vi "Receiver_3.vi"() -> ()   [LabVIEW 2013]
uses:
  <vilib>/imath/engines/lvmath/Plug In/_Char/NIMS_CH_character datatype.ctl
  <vilib>/imath/engines/lvmath2/RunTimeEngine/NodeEndStatement/NIMS_NodeEndStatement_Output.vi
  <instcachedir>/0/NIMS_NodeEndStatement_Output_53EC0D466D134D7ABD903AC30B43404B.lvgen/NIMS_NodeEndStatement_Output_53EC0D466D134D7ABD903AC30B43404B_005.vi
  <vilib>/imath/engines/lvmath2/RunTimeEngine/ErrorHandling/NIMS_Finalize Error.vi
  <vilib>/imath/engines/lvmath2/RunTimeEngine/Managers/WorkSpace/UID Generator.vi
  <vilib>/imath/engines/lvmath2/RunTimeEngine/Managers/SymbolTable/Clear UID.vi
  <instcachedir>/0/NIMS_NodeEndStatement_Output_53EC0D466D134D7ABD903AC30B43404B.lvgen/NIMS_NodeEndStatement_Output_53EC0D466D134D7ABD903AC30B43404B_011.vi
  <instcachedir>/0/NIMS_NodeEndStatement_Output_53EC0D466D134D7ABD903AC30B43404B.lvgen/NIMS_NodeEndStatement_Output_53EC0D466D134D7ABD903AC30B43404B_000.vi
  <vilib>/imath/engines/lvmath2/RunTimeEngine/BuiltInFunctions/close/NIMS_close(Enums).vi
  LabVIEW Data/MathScriptVIs/MCStatic_31879994332_6309011b735c7d3bdc345e9dbe068425.vi
  <instcachedir>/0/MCStatic_31879994332_6309011b735c7d3bdc345e9dbe068425_26C83AF4E6B94C66802D7F534C05881C.lvgen/MCStatic_31879994332_6309011b735c7d3bdc345e9dbe068425_26C83AF4E6B94C66802D7F534C05881C_000.vi
  <vilib>/imath/engines/lvmath2/RunTimeEngine/BuiltInFunctions/numelements/NIMS_numelements.vi
  <instcachedir>/0/NIMS_numelements_A776DA77F73142F68C2F209B523114C5.lvgen/NIMS_numelements_A776DA77F73142F68C2F209B523114C5_003.vi
  LabVIEW Data/MathScriptVIs/MCStatic_31879994332_e0c6d33342fcfeb52dca76011519375f.vi
  <instcachedir>/0/MCStatic_31879994332_e0c6d33342fcfeb52dca76011519375f_339AF80C0AAC43069D5B64E593FFC926.lvgen/MCStatic_31879994332_e0c6d33342fcfeb52dca76011519375f_339AF80C0AAC43069D5B64E593FFC926_000.vi
  <vilib>/imath/engines/lvmath2/RunTimeEngine/BuiltInFunctions/imag/NIMS_imag(Complex).vi
  <instcachedir>/0/NIMS_imag(Complex)_3180D40D00C843A49C2B33397F857BF3.lvgen/NIMS_imag(Complex)_3180D40D00C843A49C2B33397F857BF3_002.vi
  <vilib>/imath/engines/lvmath2/RunTimeEngine/BuiltInFunctions/figure/NIMS_figure(I32).vi
  <vilib>/imathl/engines/lvmath/Functions/Error Handling/Create Error.vi
  <vilib>/imath/engines/lvmath/Plug In/_Char/NIMS_CH_Character RV to String.vi
  <vilib>/imath/engines/lvmath2/RunTimeEngine/IndexRead/NIMS V(R2).vi
  <instcachedir>/0/NIMS V(R2)_C76619605A0E4E9F8B2FA9389712AC47.lvgen/NIMS V(R2)_C76619605A0E4E9F8B2FA9389712AC47_000.vi
  <vilib>/imath/engines/lvmath2/RunTimeEngine/ArithmeticOperatorToken/NIMS_ArithmeticOperator_plus.vi
  <instcachedir>/0/NIMS_ArithmeticOperator_plus_8A46DAFC24D445C9B2C97B626139369E.lvgen/NIMS_ArithmeticOperator_plus_8A46DAFC24D445C9B2C97B626139369E_005.vi
  <vilib>/imath/engines/lvmath2/RunTimeEngine/BuiltInFunctions/plot/NIMS_plot(G, Str).vi
  <instcachedir>/0/NIMS_plot(G, Str)_30D49D8623E0484DBD39D394DDFCBE95.lvgen/NIMS_plot(G, Str)_30D49D8623E0484DBD39D394DDFCBE95_001.vi
  <vilib>/imath/engines/lvmath2/RunTimeEngine/ErrorHandling/NIMS_Create Error From Enums.vi
  <vilib>/imath/engines/lvmath2/RunTimeEngine/BuiltInFunctions/grid/NIMS_grid(Enums).vi
  <vilib>/imath/engines/lvmath/Plug In/_Char/NIMS_CH_Character 1D to U8 1D.vi
  <vilib>/imath/engines/lvmath2/RunTimeEngine/BuiltInFunctions/plot/NIMS_plot(G, Arb).vi
  <instcachedir>/0/NIMS_plot(G, Arb)_C3943409FB664E118D06A85D9C4CA97C.lvgen/NIMS_plot(G, Arb)_C3943409FB664E118D06A85D9C4CA97C_000.vi
  <vilib>/imath/engines/lvmath2/RunTimeEngine/BuiltInFunctions/hold/NIMS_hold(Enums).vi
  <vilib>/imath/engines/lvmath2/RunTimeEngine/VariableToken/NIMS_VariableToken_CondDefined.vi
  <instcachedir>/0/NIMS_VariableToken_CondDefined_9DC5CEC47F8146B087FA2781C705B229.lvgen/NIMS_VariableToken_CondDefined_9DC5CEC47F8146B087FA2781C705B229_003.vi
  <vilib>/imath/engines/lvmath/Functions/Error Handling/MergeErrorsWrapper.vi
  <instcachedir>/0/NIMS_NodeEndStatement_Output_53EC0D466D134D7ABD903AC30B43404B.lvgen/NIMS_NodeEndStatement_Output_53EC0D466D134D7ABD903AC30B43404B_001.vi
  LabVIEW Data/MathScriptVIs/MCStatic_31879994332_4a1719067c7d5a83f01437ef7afed563.vi
  <instcachedir>/0/MCStatic_31879994332_4a1719067c7d5a83f01437ef7afed563_594FF1B2330943F592931CE525BA3D62.lvgen/MCStatic_31879994332_4a1719067c7d5a83f01437ef7afed563_594FF1B2330943F592931CE525BA3D62_001.vi
  <vilib>/imath/engines/lvmath2/RunTimeEngine/BuiltInFunctions/crosscorr/NIMS_crosscorr(GM,GM,Str).vi
  <instcachedir>/0/NIMS_crosscorr(GM,GM,Str)_C0B084FC02374B5995655F2C6E77F5A9.lvgen/NIMS_crosscorr(GM,GM,Str)_C0B084FC02374B5995655F2C6E77F5A9_001.vi
  <vilib>/imath/engines/lvmath2/RunTimeEngine/BuiltInFunctions/abs/NIMS_abs(signed).vi
  <instcachedir>/0/NIMS_abs(signed)_C4FCB8E6058B49B797C7C8D53CA5F6EC.lvgen/NIMS_abs(signed)_C4FCB8E6058B49B797C7C8D53CA5F6EC_003.vi
  <instcachedir>/0/NIMS_plot(G, Str)_30D49D8623E0484DBD39D394DDFCBE95.lvgen/NIMS_plot(G, Str)_30D49D8623E0484DBD39D394DDFCBE95_004.vi
  <instcachedir>/0/NIMS_plot(G, Str)_30D49D8623E0484DBD39D394DDFCBE95.lvgen/NIMS_plot(G, Str)_30D49D8623E0484DBD39D394DDFCBE95_005.vi
  <instcachedir>/0/NIMS_crosscorr(GM,GM,Str)_C0B084FC02374B5995655F2C6E77F5A9.lvgen/NIMS_crosscorr(GM,GM,Str)_C0B084FC02374B5995655F2C6E77F5A9_000.vi
  <instcachedir>/0/NIMS_abs(signed)_C4FCB8E6058B49B797C7C8D53CA5F6EC.lvgen/NIMS_abs(signed)_C4FCB8E6058B49B797C7C8D53CA5F6EC_005.vi
  <vilib>/imath/engines/lvmath2/RunTimeEngine/BuiltInFunctions/max/1 input/NIMS_max(RM).vi
  <instcachedir>/0/NIMS_max(RM)_95FF4207DE024F99B69DE66176218BBE.lvgen/NIMS_max(RM)_95FF4207DE024F99B69DE66176218BBE_000.vi
  <vilib>/imath/engines/lvmath2/RunTimeEngine/BuiltInFunctions/length/NIMS_length(GV).vi
  <instcachedir>/0/NIMS_length(GV)_08A3D13377FD4E4B96F5795FBF3698FA.lvgen/NIMS_length(GV)_08A3D13377FD4E4B96F5795FBF3698FA_001.vi
  <vilib>/imath/engines/lvmath2/RunTimeEngine/BuiltInFunctions/length/NIMS_length(GM).vi
  <instcachedir>/0/NIMS_length(GM)_47CEC356FCE0482D9BA47DC61C99F2C7.lvgen/NIMS_length(GM)_47CEC356FCE0482D9BA47DC61C99F2C7_005.vi
  <instcachedir>/0/NIMS V(R2)_C76619605A0E4E9F8B2FA9389712AC47.lvgen/NIMS V(R2)_C76619605A0E4E9F8B2FA9389712AC47_001.vi
  <vilib>/imath/engines/lvmath2/RunTimeEngine/RunTimeType/NIMS_RunTimeType_From StrictType (excl LVString).vi
  <instcachedir>/0/NIMS_RunTimeType_From StrictType (excl LVString)_4DEE718D6EB74582AA20236969C084FC.lvgen/NIMS_RunTimeType_From StrictType (excl LVString)_4DEE718D6EB74582AA20236969C084FC_000.vi
  <vilib>/imath/engines/lvmath2/RunTimeEngine/LocalVariableDefStatement/MC_LocalVariableDefStatement_Display.vi
  <vilib>/imath/engines/lvmath2/RunTimeEngine/BuiltInFunctions/linramp/NIMS_linramp.vi
  <instcachedir>/0/NIMS_abs(signed)_C4FCB8E6058B49B797C7C8D53CA5F6EC.lvgen/NIMS_abs(signed)_C4FCB8E6058B49B797C7C8D53CA5F6EC_006.vi
  <vilib>/imath/engines/lvmath2/RunTimeEngine/BuiltInFunctions/max/1 input/NIMS_max(RV).vi
  <instcachedir>/0/NIMS_max(RV)_237633DB1D604D5BA7001287DF3C7957.lvgen/NIMS_max(RV)_237633DB1D604D5BA7001287DF3C7957_000.vi
  <vilib>/imath/engines/lvmath2/RunTimeEngine/BuiltInFunctions/zeros/NIMS_V=zeros(I32,I32).vi
  <vilib>/imath/engines/lvmath2/RunTimeEngine/RangeToken/NIMS_Range_R2 - Integer.vi
  <instcachedir>/0/NIMS_Range_R2 - Integer_C51C130E5EA5464EA148B28CDAB9615A.lvgen/NIMS_Range_R2 - Integer_C51C130E5EA5464EA148B28CDAB9615A_000.vi
  <vilib>/imath/engines/lvmath2/RunTimeEngine/CommandStatement/MC_CommandStatement_break.vi
  <vilib>/imath/engines/lvmath2/RunTimeEngine/IndexRead/NIMS V(S).vi
  <instcachedir>/0/NIMS V(S)_0488751826AF41519A22953C041130DC.lvgen/NIMS V(S)_0488751826AF41519A22953C041130DC_005.vi
  <instcachedir>/0/NIMS_abs(signed)_C4FCB8E6058B49B797C7C8D53CA5F6EC.lvgen/NIMS_abs(signed)_C4FCB8E6058B49B797C7C8D53CA5F6EC_002.vi
  LabVIEW Data/MathScriptVIs/MCStatic_31879994332_56053b3087a32285ab019b20dd55a053.vi
  <instcachedir>/0/MCStatic_31879994332_56053b3087a32285ab019b20dd55a053_ABD68300304F468FBDE6379C6945ADEA.lvgen/MCStatic_31879994332_56053b3087a32285ab019b20dd55a053_ABD68300304F468FBDE6379C6945ADEA_000.vi
  <vilib>/imath/engines/lvmath2/RunTimeEngine/IndexReplace/NIMS V(S)=S.vi
  <instcachedir>/0/NIMS V(S)=S_66A18068148B4981A312229A93EA5C06.lvgen/NIMS V(S)=S_66A18068148B4981A312229A93EA5C06_001.vi
  LabVIEW Data/MathScriptVIs/MCStatic_31879994332_59775c3ea1da542a74dd2e471b583196.vi
  <instcachedir>/0/MCStatic_31879994332_59775c3ea1da542a74dd2e471b583196_003FAE1D6247465EB97E783626A83D88.lvgen/MCStatic_31879994332_59775c3ea1da542a74dd2e471b583196_003FAE1D6247465EB97E783626A83D88_001.vi
  <instcachedir>/0/NIMS V(S)=S_66A18068148B4981A312229A93EA5C06.lvgen/NIMS V(S)=S_66A18068148B4981A312229A93EA5C06_000.vi
  <instcachedir>/0/NIMS V(S)_0488751826AF41519A22953C041130DC.lvgen/NIMS V(S)_0488751826AF41519A22953C041130DC_000.vi
  <instcachedir>/0/NIMS_plot(G, Str)_30D49D8623E0484DBD39D394DDFCBE95.lvgen/NIMS_plot(G, Str)_30D49D8623E0484DBD39D394DDFCBE95_000.vi
  <vilib>/imath/engines/lvmath2/RunTimeEngine/BuiltInFunctions/title/NIMS_title.vi
  <instcachedir>/0/NIMS_NodeEndStatement_Output_53EC0D466D134D7ABD903AC30B43404B.lvgen/NIMS_NodeEndStatement_Output_53EC0D466D134D7ABD903AC30B43404B_012.vi
  <vilib>/imath/engines/lvmath2/RunTimeEngine/VariableToken/NIMS_VariableToken_CondDefinedDefinedByReplace.vi
  <instcachedir>/0/NIMS_VariableToken_CondDefinedDefinedByReplace_D162CFFC24174562A9FEA619A91E1A56.lvgen/NIMS_VariableToken_CondDefinedDefinedByReplace_D162CFFC24174562A9FEA619A91E1A56_002.vi
  <vilib>/imath/engines/lvmath2/RunTimeEngine/IndexRead/NIMS M(S).vi
  <instcachedir>/0/NIMS M(S)_B826C018497E4940AE96BD27B540B6FB.lvgen/NIMS M(S)_B826C018497E4940AE96BD27B540B6FB_004.vi
  <instcachedir>/0/NIMS_VariableToken_CondDefined_9DC5CEC47F8146B087FA2781C705B229.lvgen/NIMS_VariableToken_CondDefined_9DC5CEC47F8146B087FA2781C705B229_004.vi
  <vilib>/imath/engines/lvmath2/RunTimeEngine/BuiltInFunctions/min/1 input/NIMS_min(RV).vi
  <instcachedir>/0/NIMS_min(RV)_EE2DD3E2888846108C5160A664B67832.lvgen/NIMS_min(RV)_EE2DD3E2888846108C5160A664B67832_000.vi
  <vilib>/imath/engines/lvmath2/RunTimeEngine/IndexRead/NIMS M(S,S).vi
  <instcachedir>/0/NIMS M(S,S)_AC51E74150A542F7991B9634C66F3096.lvgen/NIMS M(S,S)_AC51E74150A542F7991B9634C66F3096_003.vi
  <vilib>/imath/engines/lvmath2/RunTimeEngine/RowToken/NIMS_RowToken_M_SorRV.vi
  <instcachedir>/0/NIMS_RowToken_M_SorRV_6464340A296F47B6970F468C8541F43A.lvgen/NIMS_RowToken_M_SorRV_6464340A296F47B6970F468C8541F43A_001.vi
  <vilib>/imath/engines/lvmath2/RunTimeEngine/IndexReplace/NIMS M($,S)=M.vi
  <instcachedir>/0/NIMS M($,S)=M_9C9B00E4835C49429FADE7516194B3E0.lvgen/NIMS M($,S)=M_9C9B00E4835C49429FADE7516194B3E0_002.vi
  <vilib>/imath/engines/lvmath2/RunTimeEngine/IndexReplace/NIMS M($,S)=V.vi
  <instcachedir>/0/NIMS M($,S)=V_D41FDDDB142B47FCA5EF37B60D4970ED.lvgen/NIMS M($,S)=V_D41FDDDB142B47FCA5EF37B60D4970ED_001.vi
  <vilib>/imath/engines/lvmath2/RunTimeEngine/ArithmeticOperatorToken/NIMS_ArithmeticOperator_minus.vi
  <instcachedir>/0/NIMS_ArithmeticOperator_minus_5462A7974F41415E96B34B7C9D041F4F.lvgen/NIMS_ArithmeticOperator_minus_5462A7974F41415E96B34B7C9D041F4F_001.vi
  <vilib>/imath/engines/lvmath2/RunTimeEngine/BuiltInFunctions/sum/NIMS_sum(GM,Sca).vi
  <instcachedir>/0/NIMS_sum(GM,Sca)_6844B20AF95244A89239C08EE60A7865.lvgen/NIMS_sum(GM,Sca)_6844B20AF95244A89239C08EE60A7865_001.vi
  <vilib>/imath/engines/lvmath2/RunTimeEngine/BuiltInFunctions/crosscorr/NIMS_crosscorr(GM,Sca,Str).vi
  <instcachedir>/0/NIMS_crosscorr(GM,Sca,Str)_6201EFE436AF4A49A2EDE7F536F431B0.lvgen/NIMS_crosscorr(GM,Sca,Str)_6201EFE436AF4A49A2EDE7F536F431B0_000.vi
  <instcachedir>/0/NIMS_length(GV)_08A3D13377FD4E4B96F5795FBF3698FA.lvgen/NIMS_length(GV)_08A3D13377FD4E4B96F5795FBF3698FA_002.vi
  MATLAB_func/RX_RRC_filtering.m
  MATLAB_func/rtrcpulse.m
  MATLAB_func/gardner_symbol_recovery.m
  MATLAB_func/b2_16qam.m
  MATLAB_func/frequency_synchronisation_sample.m
  MATLAB_func/phase_synchronisation_sample.m
  <vilib>/imath/engines/lvmath2/RunTimeEngine/Managers/SymbolTable/NIMS_WorkSpace.lvlib
panel:
  out "error":dbl[](array[numeric])
  out "signal_out":i32[][](array[numeric])
  out "Real 2":dbl
  out "N":i32
  out "L":i32
  out "Symbols 4":cdb[](graph)
  out "1-D Array of Complex":cdb[](array[numeric])
  out "wave array":cdb[](array[numeric])
  out "sym array":cdb[](array[numeric])
  out "Symbols 3":cdb[](graph)
  out "1-D Array of Complex 4":cdb[](array[numeric])
  out "Real":dbl
  out "Waveform Chart":dbl[](graph)
  out "First Start":dbl(graph)
  out "Symbols 1":cdb[](graph)
  out "Symbols 2":cdb[](graph)
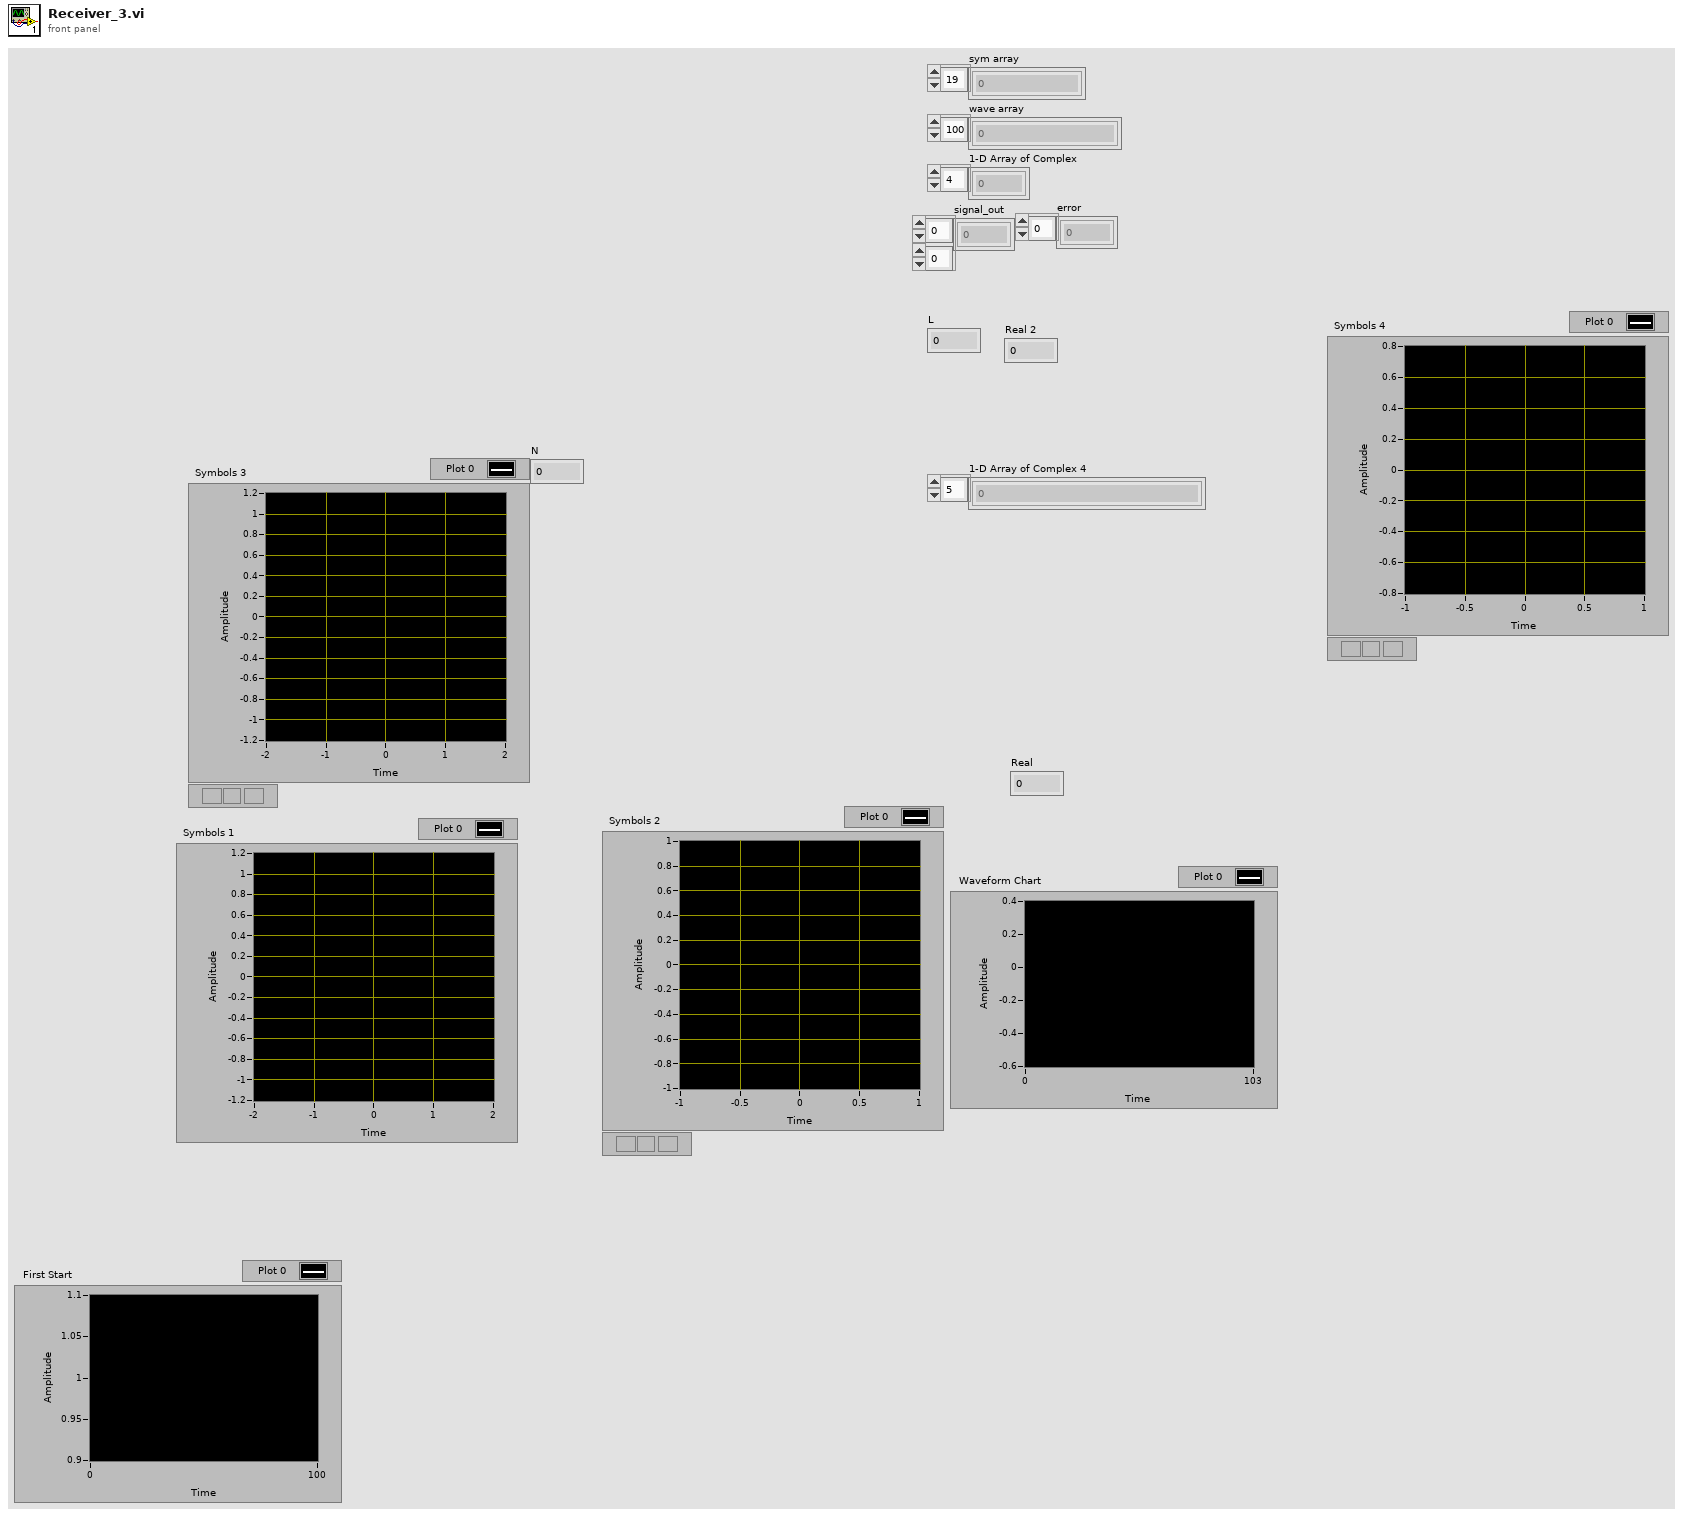
[diagram p1: front panel]
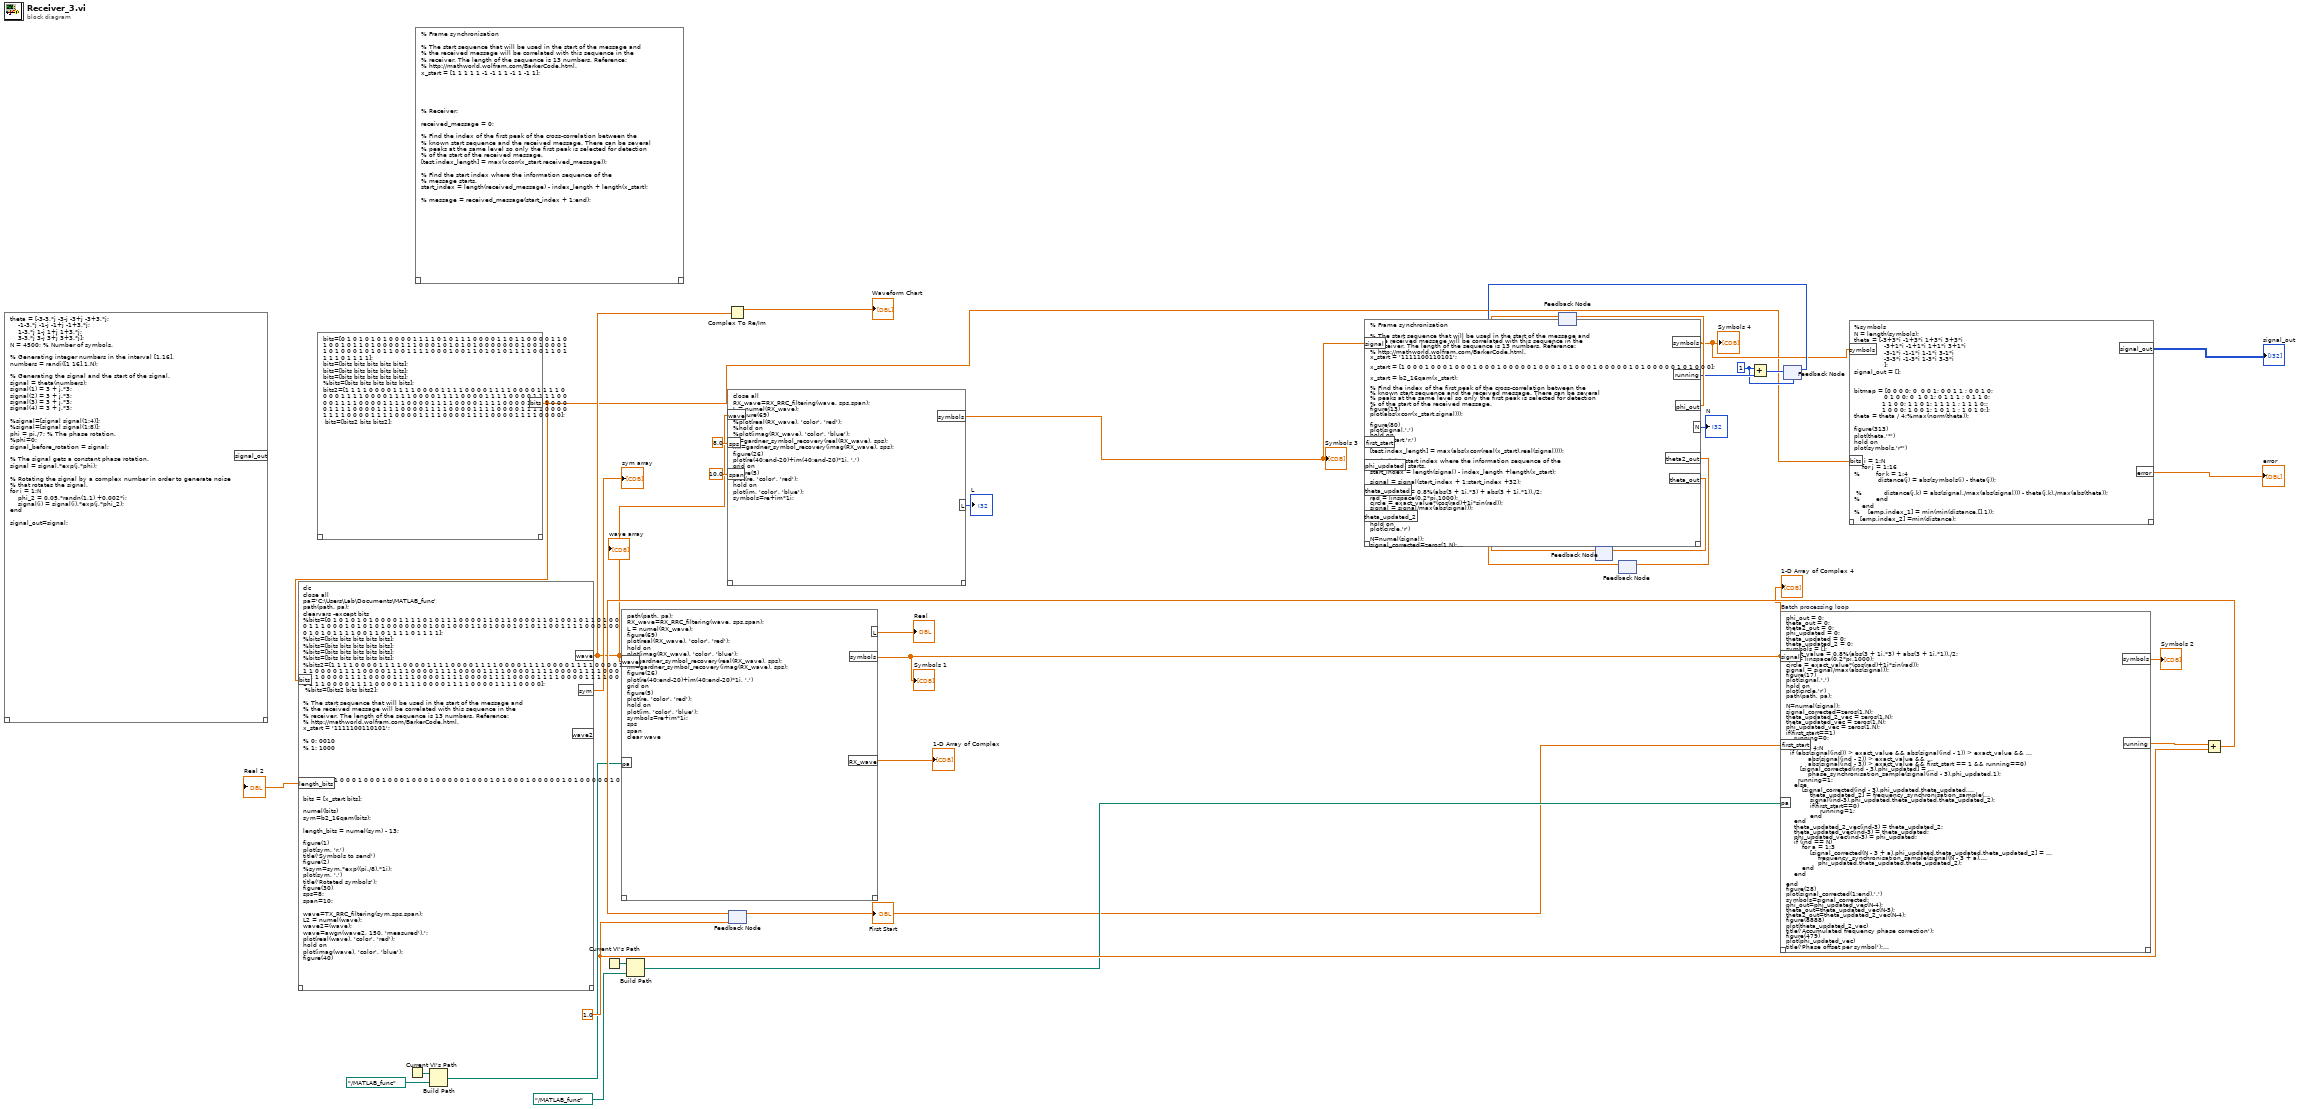
[diagram p0: block diagram]
diagram:
  w9 = 1 ("x")
  w36 = 1.0
  n1 = script code="theta = [-3-3.*j -3-j -3+j -3+3.*j;\n    -1-3.*j -1-j -1+j -1+3.*j;\n    1-3.*j 1-j 1+j 1+3.*j;\n    3-3.*j 3-j 3+j 3+3.*j];\nN = 4500; % Number of symbols.\n\n% Generating integer numbers in the interval [1,16].\nnumbers = randi([1 16],1,N);\n\n% Generating the signal and the start of the signal.\nsignal = theta(numbers);\nsignal(1) = 3 + j.*3;\nsignal(2) = 3 + j.*3;\nsignal(3) = 3 + j.*3;\nsignal(4) = 3 + j.*3;\n\n%signal=[signal signal(1:4)];\n%signal=[signal signal(1:8)];\nphi = pi./7; % The phase rotation.\n%phi=0;\nsignal_before_rotation = signal;\n\n% The signal gets a constant phase rotation.\nsignal = signal.*exp(j.*phi);\n\n% Rotating the signal by a complex number in order to generate noise\n% that rotates the signal.\nfor i = 1:N\n    phi_2 = 0.05.*randn(1,1) +0.002*i;\n    signal(i) = signal(i).*exp(j.*phi_2);\nend\n\nsignal_out=signal;"() -> ()  [unwired: 1 in, 2 out]
  n2 = mathscript code="bits=[0 1 0 1 0 1 0 1 0 0 0 0 1 1 1 1 0 1 0 1 1 1 0 0 0 0 1 1 0 1 1 0 0 0 0 1 1 0 1 0 0 1 0 1 1 0 1 0 0 0 0 1 1 1 0 0 0 1 0 1 0 1 0 1 0 0 0 0 0 0 0 1 0 0 1 0 0 0 1 1 0 1 0 0 0 1 0 1 0 1 1 0 0 1 1 1 1 0 0 0 1 0 0 1 1 0 1 0 1 0 1 1 1 1 0 0 1 1 0 1 1 1 1 0 1 1 1 1];\nbits=[bits bits bits bits bits];\nbits=[bits bits bits bits bits];\nbits=[bits bits bits bits bits];\n%bits=[bits bits bits bits bits];\nbits2=[1 1 1 1 0 0 0 0 1 1 1 1 0 0 0 0 1 1 1 1 0 0 0 0 1 1 1 1 0 0 0 0 1 1 1 1 0 0 0 0 1 1 1 1 0 0 0 0 1 1 1 1 0 0 0 0 1 1 1 1 0 0 0 0 1 1 1 1 0 0 0 0 1 1 1 1 0 0 0 0 1 1 1 1 0 0 0 0 1 1 1 1 0 0 0 0 1 1 1 1 0 0 0 0 1 1 1 1 0 0 0 0 1 1 1 1 0 0 0 0 1 1 1 1 0 0 0 0 1 1 1 1 0 0 0 0 1 1 1 1 0 0 0 0 1 1 1 1 0 0 0 0 1 1 1 1 0 0 0 0 1 1 1 1 0 0 0 0 1 1 1 1 0 0 0 0 1 1 1 1 0 0 0 0 1 1 1 1 0 0 0 0 1 1 1 1 0 0 0 0]; \n bits=[bits2 bits bits2];"() -> ("bits"=w2:dbl[])  [unwired: 1 in, 1 out]
  n3 = script code="clc\nclose all\npa='C:\\Users\\Lab\\Documents\\MATLAB_func'\npath(path, pa);\nclearvars -except bits\n%bits=[0 1 0 1 0 1 0 1 0 0 0 0 1 1 1 1 0 1 0 1 1 1 0 0 0 0 1 1 0 1 1 0 0 0 0 1 1 0 1 0 0 1 0 1 1 0 1 0 0 0 0 1 1 1 0 0 0 1 0 1 0 1 0 1 0 0 0 0 0 0 0 1 0 0 1 0 0 0 1 1 0 1 0 0 0 1 0 1 0 1 1 0 0 1 1 1 1 0 0 0 1 0 0 1 1 0 1 0 1 0 1 1 1 1 0 0 1 1 0 1 1 1 1 0 1 1 1 1];\n%bits=[bits bits bits bits bits];\n%bits=[bits bits bits bits bits];\n%bits=[bits bits bits bits bits];\n%bits=[bits bits bits bits bits];\n%bits2=[1 1 1 1 0 0 0 0 1 1 1 1 0 0 0 0 1 1 1 1 0 0 0 0 1 1 1 1 0 0 0 0 1 1 1 1 0 0 0 0 1 1 1 1 0 0 0 0 1 1 1 1 0 0 0 0 1 1 1 1 0 0 0 0 1 1 1 1 0 0 0 0 1 1 1 1 0 0 0 0 1 1 1 1 0 0 0 0 1 1 1 1 0 0 0 0 1 1 1 1 0 0 0 0 1 1 1 1 0 0 0 0 1 1 1 1 0 0 0 0 1 1 1 1 0 0 0 0 1 1 1 1 0 0 0 0 1 1 1 1 0 0 0 0 1 1 1 1 0 0 0 0 1 1 1 1 0 0 0 0 1 1 1 1 0 0 0 0 1 1 1 1 0 0 0 0 1 1 1 1 0 0 0 0 1 1 1 1 0 0 0 0 1 1 1 1 0 0 0 0]; \n %bits=[bits2 bits bits2];\n\n% The start sequence that will be used in the start of the message and\n% the received message will be correlated with this sequence in the \n% receiver. The length of the sequence is 13 numbers. Reference: \n% http://mathworld.wolfram.com/BarkerCode.html.\nx_start = '1111100110101';\n\n% 0: 0010\n% 1: 1000\n\n\n\n\nx_start = [1 0 0 0 1 0 0 0 1 0 0 0 1 0 0 0 1 0 0 0 0 0 1 0 0 0 1 0 1 0 0 0 1 0 0 0 0 0 1 0 1 0 0 0 0 0 1 0 1 0 0 0];\n\nbits = [x_start bits];\n\nnumel(bits)\nsym=b2_16qam(bits);\n\nlength_bits = numel(sym) - 13;\n\nfigure(1)\nplot(sym, 'r.')\ntitle('Symbols to send')\nfigure(2)\n%sym=sym.*exp((pi./8).*1i);\nplot(sym, '.')\ntitle('Rotated symbols');\nfigure(30)\nsps=8;\nspan=10;\n\nwave=TX_RRC_filtering(sym,sps,span);\nL2 = numel(wave);\nwave2=(wave);\nwave=awgn(wave2, 150, 'measured').';\nplot(real(wave), 'color', 'red');\nhold on\nplot(imag(wave), 'color', 'blue');\nfigure(40)"("bits"=w2) -> ("wave"=w19:cdb[], "sym"=→"sym array":cdb[], "length_bits"=→"Real 2":dbl)  [unwired: 1 in, 2 out]
  "wave array" <- w19
  n4 = Current VI's Path() -> (path=w29:path)
  n5 = mathscript code="% Frame synchronisation\n\n% The start sequence that will be used in the start of the message and\n% the received message will be correlated with this sequence in the \n% receiver. The length of the sequence is 13 numbers. Reference: \n% http://mathworld.wolfram.com/BarkerCode.html.\nx_start = [1 1 1 1 1 -1 -1 1 1 -1 1 -1 1];\n\n\n\n\n\n% Receiver:\n\nreceived_message = 0;\n\n% Find the index of the first peak of the cross-correlation between the \n% known start sequence and the received message. There can be several \n% peaks at the same level so only the first peak is selected for detection \n% of the start of the received message.\n[test,index_length] = max(xcorr(x_start,received_message));\n\n% Find the start index where the information sequence of the \n% message starts.\nstart_index = length(received_message) - index_length + length(x_start);\n\n% message = received_message(start_index + 1:end);"() -> ()  [unwired: 1 in, 1 out]
  n6 = Build Path(base path=w29, name or relative path=path "../MATLAB_func") -> (appended path=w30:path)
  n7 = Current VI's Path() -> (path=w33:path)
  n8 = script code="path(path, pa);\nRX_wave=RX_RRC_filtering(wave, sps,span);\nL = numel(RX_wave);\nfigure(69)\nplot(real(RX_wave), 'color', 'red');\nhold on\nplot(imag(RX_wave), 'color', 'blue');\nre=gardner_symbol_recovery(real(RX_wave), sps);\nim=gardner_symbol_recovery(imag(RX_wave), sps);\nfigure(26)\nplot(re(40:end-20)+im(40:end-20)*1i, '.')\ngrid on\nfigure(5)\nplot(re, 'color', 'red');\nhold on\nplot(im, 'color', 'blue');\nsymbols=re+im*1i;\nsps\nspan\nclear wave"("wave"=w19, "pa"=w30) -> ("symbols"=w22:cdb[], "L"=→"Real":dbl, "RX_wave"=→"1-D Array of Complex":cdb[])  [unwired: 1 in, 1 out]
  "Symbols 1" <- w22
  "1-D Array of Complex 4" <- w22
  n9 = Build Path(base path=w33, name or relative path=path "../MATLAB_func") -> (appended path=w34:path)
  n10 = mathscript code="close all\nRX_wave=RX_RRC_filtering(wave, sps,span);\nL = numel(RX_wave);\n%figure(69)\n%plot(real(RX_wave), 'color', 'red');\n%hold on\n%plot(imag(RX_wave), 'color', 'blue');\nre=gardner_symbol_recovery(real(RX_wave), sps);\nim=gardner_symbol_recovery(imag(RX_wave), sps);\nfigure(26)\nplot(re(40:end-20)+im(40:end-20)*1i, '.')\ngrid on\nfigure(5)\nplot(re, 'color', 'red');\nhold on\nplot(im, 'color', 'blue');\nsymbols=re+im*1i;"("wave"=w19, "sps"=8.0, "span"=10.0) -> ("symbols"=w18:cdb[], "L"=→"L":i32)  [unwired: 1 in, 1 out]
  "Symbols 3" <- w18
  n11 = Complex To Re/Im(x + iy=w19) -> (x=→"Waveform Chart":dbl[])  [unwired: 1 out]
  n12 = feedback #1(w36) -> (w25:dbl)
  "First Start" <- w25
  n13 = feedback #2() -> (w12:dbl)  [unwired: 1 in]
  n14 = feedback #3() -> (w16:dbl)  [unwired: 1 in]
  n15 = feedback #4() -> (w14:dbl)  [unwired: 1 in]
  n16 = script code="phi_out = 0;\ntheta_out = 0;\ntheta2_out = 0;\nphi_updated = 0;\ntheta_updated = 0;\ntheta_updated_2 = 0;\nsymbols = [];\nexact_value = 0.8%(abs(3 + 1i.*3) + abs(3 + 1i.*1))./2;\nrad = linspace(0,2*pi,1000);\ncircle = exact_value*(cos(rad)+1i*sin(rad));\nsignal = signal/max(abs(signal));\nfigure(17)\nplot(signal,'.')\nhold on\nplot(circle,'r')\npath(path, pa);\n\nN=numel(signal);\nsignal_corrected=zeros(1,N);\ntheta_updated_2_vec = zeros(1,N);\ntheta_updated_vec = zeros(1,N);\nphi_updated_vec = zeros(1,N);\nif(first_start==1)\n    running=0;\nend\nfor ind= 4:N\n  if (abs(signal(ind)) > exact_value && abs(signal(ind - 1)) > exact_value && ...\n           abs(signal(ind - 2)) > exact_value && ...\n           abs(signal(ind - 3)) > exact_value && first_start == 1 && running==0)\n       [signal_corrected(ind - 3),phi_updated] = ...\n           phase_synchronisation_sample(signal(ind - 3),phi_updated,1);\n      running=1;\n    else\n        [signal_corrected(ind - 3),phi_updated,theta_updated,...\n            theta_updated_2] = frequency_synchronisation_sample(...\n            signal(ind-3),phi_updated,theta_updated,theta_updated_2);\n            if(first_start==0)\n                 running=1;\n            end\n    end\n    theta_updated_2_vec(ind-3) = theta_updated_2;\n    theta_updated_vec(ind-3) = theta_updated;\n    phi_updated_vec(ind-3) = phi_updated;\n    if (ind == N)\n        for a = 1:3\n            [signal_corrected(N - 3 + a),phi_updated,theta_updated,theta_updated_2] = ...\n                frequency_synchronisation_sample(signal(N - 3 + a),...\n                phi_updated,theta_updated,theta_updated_2);\n        end\n    end\n\nend\nfigure(28)\nplot(signal_corrected(1:end),'.')\nsymbols=signal_corrected;\nphi_out=phi_updated_vec(N-4);\ntheta_out=theta_updated_vec(N-5);\ntheta2_out=theta_updated_2_vec(N-4);\nfigure(8888)\nplot(theta_updated_2_vec)\ntitle('Accumulated frequency phase correction');\nfigure(479)\nplot(phi_updated_vec)\ntitle('Phase offset per symbol');\nhold off\nfigure(1337)\nplot(symbols(100:end-20),'.')\nclear all\n% clearvars -except symbols running phi_out theta_out theta2_out" "Batch processing loop"("signal"=w22, "first_start"=w25, "pa"=w34) -> ("symbols"=→"Symbols 2":cdb[], "running"=w31:dbl)  [unwired: 1 in, 1 out]
  n17 = feedback #5(w9) -> (w8:i32)
  n18 = mathscript code="% Frame synchronisation\n\n% The start sequence that will be used in the start of the message and\n% the received message will be correlated with this sequence in the \n% receiver. The length of the sequence is 13 numbers. Reference: \n% http://mathworld.wolfram.com/BarkerCode.html.\nx_start = '1111100110101';\n\nx_start = [1 0 0 0 1 0 0 0 1 0 0 0 1 0 0 0 1 0 0 0 0 0 1 0 0 0 1 0 1 0 0 0 1 0 0 0 0 0 1 0 1 0 0 0 0 0 1 0 1 0 0 0];\n\nx_start = b2_16qam(x_start);\n\n% Find the index of the first peak of the cross-correlation between the \n% known start sequence and the received message. There can be several \n% peaks at the same level so only the first peak is selected for detection \n% of the start of the received message.\nfigure(13)\nplot(abs(xcorr(x_start,signal)));\n\nfigure(80)\nplot(signal,'.')\nhold on\nplot(x_start,'r.')\n\n[test,index_length] = max(abs(xcorr(real(x_start),real(signal))));\n\n% Find the start index where the information sequence of the \n% message starts.\nstart_index = length(signal) - index_length +length(x_start);\n\nsignal = signal(start_index + 1:start_index +32);\n\nexact_value = 0.8%(abs(3 + 1i.*3) + abs(3 + 1i.*1))./2;\nrad = linspace(0,2*pi,1000);\ncircle = exact_value*(cos(rad)+1i*sin(rad));\nsignal = signal/max(abs(signal));\nfigure(17)\nplot(signal,'.')\nhold on\nplot(circle,'r')\n\nN=numel(signal);\nsignal_corrected=zeros(1,N);\ntheta_updated_2_vec = zeros(1,N);\ntheta_updated_vec = zeros(1,N);\nphi_updated_vec = zeros(1,N);\nif(first_start==1)\n    running=0;\nend\nfor ind= 4:N\n  if (abs(signal(ind)) > exact_value && abs(signal(ind - 1)) > exact_value && ...\n           abs(signal(ind - 2)) > exact_value && ...\n           abs(signal(ind - 3)) > exact_value && first_start == 1 && running==0)\n       [signal_corrected(ind - 3),phi_updated] = ...\n           phase_synchronisation_sample(signal(ind - 3),phi_updated,1);\n      running=1;\n    else\n        [signal_corrected(ind - 3),phi_updated,theta_updated,...\n            theta_updated_2] = frequency_synchronisation_sample(...\n            signal(ind-3),phi_updated,theta_updated,theta_updated_2);\n            if(first_start==0)\n                 running=1;\n            end\n    end\n    theta_updated_2_vec(ind-3) = theta_updated_2;\n    theta_updated_vec(ind-3) = theta_updated;\n    phi_updated_vec(ind-3) = phi_updated;\n    if (ind == N)\n        for a = 1:3\n            [signal_corrected(N - 3 + a),phi_updated,theta_updated,theta_updated_2] = ...\n                frequency_synchronisation_sample(signal(N - 3 + a),...\n                phi_updated,theta_updated,theta_updated_2);\n        end\n    end\n\nend\nfigure(28)\nplot(signal_corrected(1:end),'.')\nsymbols=signal_corrected;\nphi_out=phi_updated_vec(N-4);\ntheta_out=theta_updated_vec(N-5);\ntheta2_out=theta_updated_2_vec(N-4);\nfigure(8888)\nplot(theta_updated_2_vec)\ntitle('Accumulated frequency phase correction');\nfigure(479)\nplot(phi_updated_vec)\ntitle('Phase offset per symbol');\nhold off\nfigure(1337)\nplot(symbols(1000:end-20),'.')"("first_start"=w8, "signal"=w18, "phi_updated"=w12, "theta_updated"=w16, "theta_updated_2"=w14) -> ("symbols"=w4:cdb[], "running"=w11:i32, "phi_out"=w13:dbl, "theta2_out"=w15:dbl, "theta_out"=w17:dbl, "N"=→"N":i32)  [unwired: 1 in, 1 out]
  "Symbols 4" <- w4
  n19 = feedback-in #2(w13) -> ()
  n20 = feedback-in #3(w17) -> ()
  n21 = feedback-in #4(w15) -> ()
  n22 = Add(x=w9, y=w11) -> (x+y=w10:i32)
  n23 = feedback-in #5(w10) -> ()
  n24 = mathscript code="%symbols\nN = length(symbols);\ntheta = [-3+3*i -1+3*i 1+3*i 3+3*i\n               -3+1*i -1+1*i 1+1*i 3+1*i\n               -3-1*i -1-1*i 1-1*i 3-1*i\n               -3-3*i -1-3*i 1-3*i 3-3*i\n               ];\nsignal_out = [];\n\n\nbitmap = [0 0 0 0; 0  0 0 1; 0 0 1 1 ; 0 0 1 0;\n               0 1 0 0; 0  1 0 1; 0 1 1 1 ; 0 1 1 0;\n              1 1 0 0; 1 1 0 1; 1 1 1 1 ; 1 1 1 0;;\n              1 0 0 0; 1 0 0 1; 1 0 1 1 ; 1 0 1 0;];\ntheta = theta / 4;%max(norm(theta));\n\nfigure(313)\nplot(theta,'*')\nhold on\nplot(symbols,'r*')\n\nfor i = 1:N\n    for j = 1:16\n%        for k = 1:4\n            distance(j) = abs(symbols(i) - theta(j));\n            \n %           distance(j,k) = abs(signal./max(abs(signal))) - theta(j,k)./max(abs(theta));\n%        end\n    end\n%    [emp,index_1] = min(min(distance,[],1));\n   [emp,index_2] =min(distance);\n    \n    signal_out = [signal_out bitmap(index_2,1) bitmap(index_2,2) bitmap(index_2,3) bitmap(index_2,4)];\nend\n\n%bits=[0 1 0 1 0 1 0 1 0 0 0 0 1 1 1 1 0 1 0 1 1 1 0 0 0 0 1 1 0 1 1 0 0 0 0 1 1 0 1 0 0 1 0 1 1 0 1 0 0 0 0 1 1 1 0 0 0 1 0 1 0 1 0 1 0 0 0 0 0 0 0 1 0 0 1 0 0 0 1 1 0 1 0 0 0 1 0 1 0 1 1 0 0 1 1 1 1 0 0 0 1 0 0 1 1 0 1 0 1 0 1 1 1 1 0 0 1 1 0 1 1 1 1 0 1 1 1 1];\n%bits=[bits bits bits bits bits];\n%bits=[bits bits bits bits bits];\n%bits=[bits bits bits bits bits];\n%bits=[bits bits bits bits bits];\n%bits2=[1 1 1 1 0 0 0 0 1 1 1 1 0 0 0 0 1 1 1 1 0 0 0 0 1 1 1 1 0 0 0 0 1 1 1 1 0 0 0 0 1 1 1 1 0 0 0 0 1 1 1 1 0 0 0 0 1 1 1 1 0 0 0 0 1 1 1 1 0 0 0 0 1 1 1 1 0 0 0 0 1 1 1 1 0 0 0 0 1 1 1 1 0 0 0 0 1 1 1 1 0 0 0 0 1 1 1 1 0 0 0 0 1 1 1 1 0 0 0 0 1 1 1 1 0 0 0 0 1 1 1 1 0 0 0 0 1 1 1 1 0 0 0 0 1 1 1 1 0 0 0 0 1 1 1 1 0 0 0 0 1 1 1 1 0 0 0 0 1 1 1 1 0 0 0 0 1 1 1 1 0 0 0 0 1 1 1 1 0 0 0 0 1 1 1 1 0 0 0 0]; \n %bits=[bits2 bits bits2];\n\ntest(:,1) = signal_out;\ntest(:,2) = bits;\nerror = sum(abs(bits - signal_out));"("symbols"=w4, "bits"=w2) -> ("signal_out"=→"signal_out":i32[][], "error"=→"error":dbl[])  [unwired: 1 in, 1 out]
  n25 = Add(x=w31, y=w36) -> (x+y=w37:dbl)
  n26 = feedback-in #1(w37) -> ()
